vi "Variant Preserve Type.vi"(7 "Variant Type":variant, 8 "error in (no error)":errorcluster, 11 "Variant in":variant) -> (0 "error out":errorcluster, 3 "Variant out":variant)   [LabVIEW 2019, in "labview_json.lvlib"]
uses:
  labview_json.lvlib
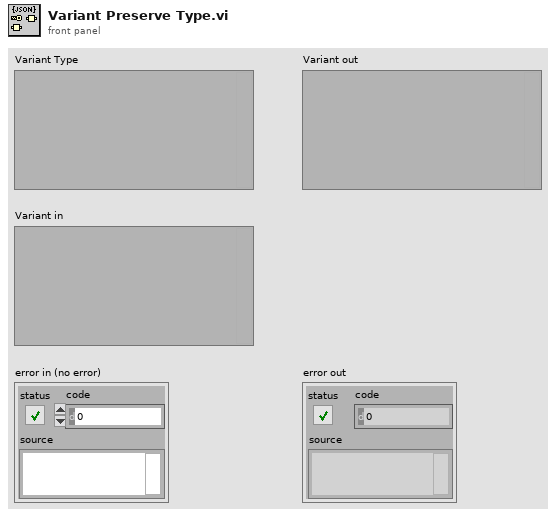
[diagram p1: front panel]
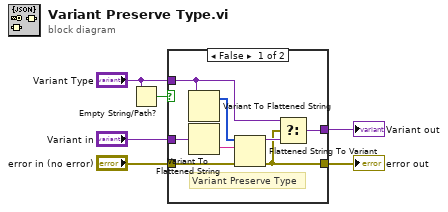
[diagram p0: block diagram]
diagram:
  n1 = Empty String/Path?(string/path="Variant Type") -> (empty?=w1:bool)
  n2 = case shown="False" w1 {
    tunnel: "error in (no error)" -> [w11 w15]
    tunnel: [w10 w15] -> w5
    tunnel: [w9 w16] -> w4
    tunnel: "Variant in" -> [w8 w16]
    tunnel: "Variant Type" -> [w7 _]
    frame False {
      # "Variant Preserve Type"
      n3 = Variant To Flattened String(Variant=w7) -> (1:w12:i16[])  [unwired: 1 out]
      n4 = Variant To Flattened String(Variant=w8) -> (data string=w14:string)  [unwired: 1 out]
      n5 = Flattened String To Variant(4:w11, 6:w14, 7:w12) -> (0:w10:errorcluster, 3:w13:variant)
      n6 = Select(t=w7, s=w10, f=w13) -> (s? t:f=w9:variant)
    }
    frame True {
      # "No variant type\nspecified, return\nvariant in"
    }
  }
  "error out" <- w5
  "Variant out" <- w4
